vi "NewAutoWriteJSONFile.vi"(9 "Array":T2[](array[typedef]), 10 "Comment":string, 11 "Trajectory File Name":path) -> (0 "error out":errorcluster)   [LabVIEW 2023]
doc: "Create a CSV file from a Trajectory data structure. This can be used on a PC or the RoboRIO.\n\nParameters:\n - Trajectory - Data structure containing trajectory\n - TrajectoryConfig - Trajectory configuration\n - Trajectory File Name - File name to write to. Existing files are overwritten.\n - Comment - Comment string to include in file comments.\n - Waypoints - waypoints to include in file comments\n - TrajectoryIsRelative - Relative if TRUE otherwise absolute\n - TrajectoryIsCubic - Cubic if TRUE otherwise Quintic\n\nReturns:\n - Error out - returned error cluster\n\nReturns:\n - outTrajectory - Trajectory data structure\n - Error out - returned error cluster"
uses:
  NewAutoStepTypedef.ctl
  NewAutoStepTypeEnum.ctl
  <vilib>/Rock Robotics/WPI/ThirdParty/JAS_Junk/TrajLib/Trajectory_Library.lvlib
panel:
  out "AutoRoutine":T1
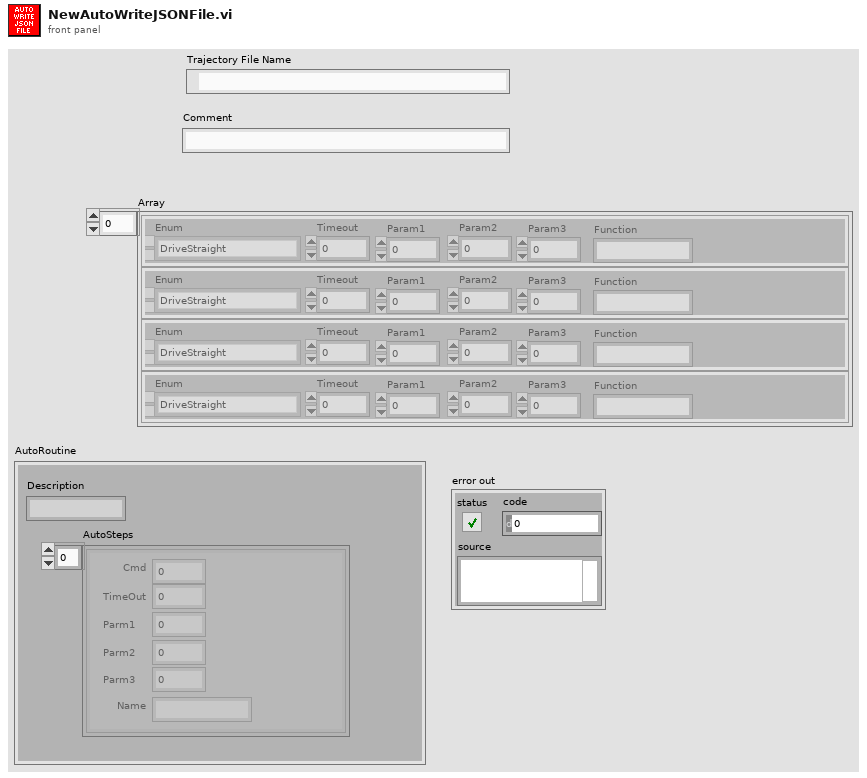
[diagram p1: front panel]
types:
  T1 = cluster{"Description":string, "AutoSteps":cluster{"Cmd":i32, "TimeOut":dbl, "Parm1":dbl, "Parm2":dbl, "Parm3":dbl, "Name":string}[]}
  T2 = typedef "NewAutoStepTypedef.ctl" = cluster{"Enum":T3, "Timeout":dbl, "Param1":dbl, "Param2":dbl, "Param3":dbl, "Function":string}
  T3 = typedef "NewAutoStepTypeEnum.ctl" = enum16{"DriveStraight", "DriveTurn", "FollowAbsoluteTrajectory", "FollowRelativeTrajectory", "AutoWait", "ElevToRest", "ElevToFloor", "ElevToSource", "ElevToL1", "ElevToL2", "ElevToL3", "ElevToL4", "ElevToAlgae1", "ElevToAlgae2", "ElevToBarge", "ElevCancel", "IntakeCoral", "IntakeAlgae", "IntakeDepositCoral", "IntakeDepositAlgae", "IntakeCancel", "ElevRestWait", "ElevFloorWait", "ElevSourceWait", "ElevL1Wait", "ElevL2Wait", "ElevAlgae1Wait", "ElevL3Wait", "ElevAlgae2Wait", "ElevL4Wait", "ElevBargeWait", "IntakeWait", "FollowAbsTrajWithTimedCmd", "FollowRelTrajWithTimedCmd"}
  T4 = cluster{"Cmd":i32, "TimeOut":dbl, "Parm1":dbl, "Parm2":dbl, "Parm3":dbl, "Name":string}
  T5 = enum16{"open", "replace", "create", "open or create", "replace or create", "replace or create with confirmation"}
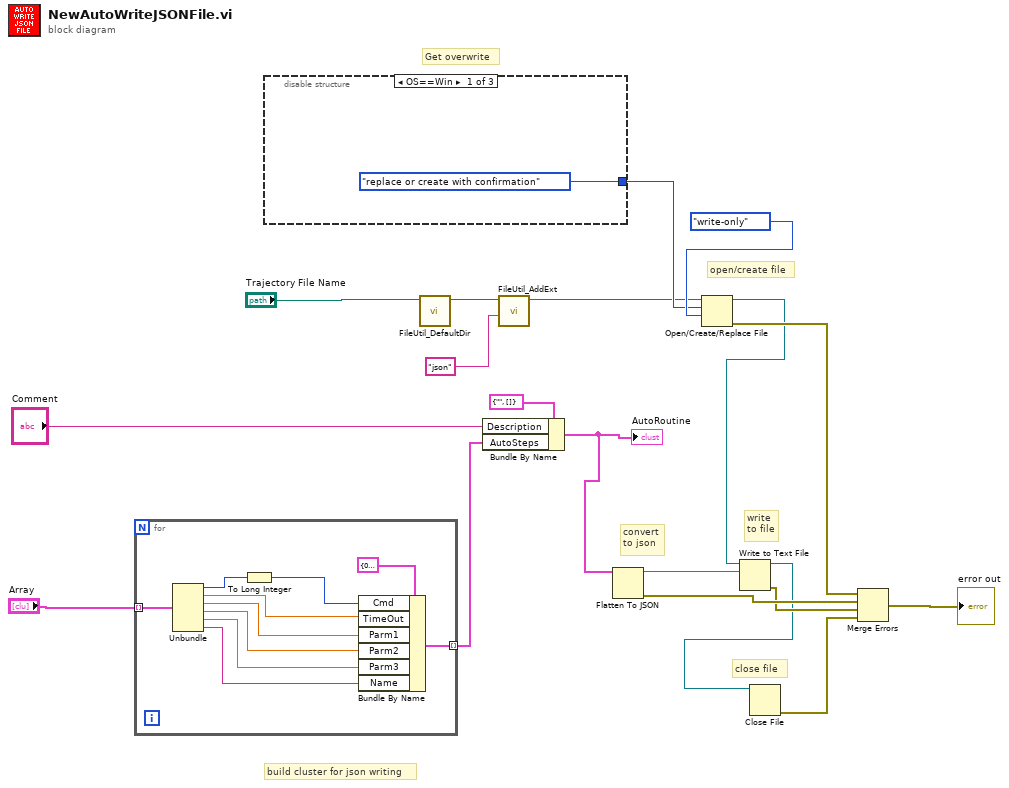
[diagram p0: block diagram]
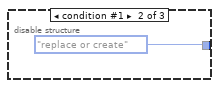
[diagram p2: hidden frame]
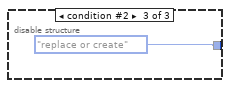
[diagram p3: hidden frame]
diagram:
  # "write\nto file"
  # "convert\nto json"
  # "build cluster for json writing"
  # "Get overwrite"
  # "open/create file"
  # "close file"
  n1 = for {
    tunnel: "Array" -> [w29] mode=indexing
    tunnel: [w20] -> w8 mode=indexing
    n2 = Unbundle(w29) -> ("Enum"=w28:T3, "Timeout"=w25:dbl, "Param1"=w24:dbl, "Param2"=w23:dbl, "Param3"=w22:dbl, "Function"=w21:string)
    n3 = To Long Integer(number=w28) -> (32bit integer=w26:i32)
    n4 = Bundle By Name(cluster=T4 {"Cmd"=0, "TimeOut"=0.0, "Parm1"=0.0, "Parm2"=0.0, "Parm3"=0.0, "Name"=""} ("AutoStep"), "Cmd"=w26, "TimeOut"=w25, "Parm1"=w24, "Parm2"=w23, "Parm3"=w22, "Name"=w21) -> (w20:T4)
  }
  n5 = disable-structure shown="OS==Win" {
    disable-tunnel: [T5."replace or create with confirmation" ("operation (0:open)") T5."replace or create" ("operation (0:open)") T5."replace or create" ("operation (0:open)")] -> w17
    frame condition #0 (active) {
    }
    frame condition #1 {
    }
    frame condition #2 {
    }
  }
  n6 = call <vilib>:"FileUtil_DefaultDir.vi"("Path in"="Trajectory File Name") -> ("Path Out"=w16:path)  [unwired: 10 in]
  n7 = Bundle By Name(cluster=T1 {"Description"="", "AutoSteps"=[]} ("AutoRoutine"), "Description"="Comment", "AutoSteps"=w8) -> (w7:T1)
  "AutoRoutine" <- w7
  n8 = call <vilib>:"FileUtil_AddExt.vi"("Extension"="json", "Path in"=w16) -> ("Path out"=w13:path)  [unwired: 9 in]
  n9 = Flatten To JSON(anything=w7) -> (JSON string=w6:string, 11:w5:errorcluster)  [unwired: 2 in]
  n10 = Open/Create/Replace File(file path (use dialog)=w13, operation (0:open)=w17, access (0:read/write)=enum16{"read/write", "read-only", "write-only"}."write-only") -> (refnum out=w9:refnum<file>, error out=w18:errorcluster)  [unwired: 3 in, 1 out]
  n11 = Write to Text File(file (use dialog)=w9, text=w6) -> (refnum out=w3:refnum<file>, error out=w4:errorcluster)  [unwired: 2 in, 1 out]
  n12 = Close File(refnum=w3) -> (error out=w2:errorcluster)  [unwired: 1 in, 1 out]
  n13 = Merge Errors(w18, w5, w4, w2) -> (→"error out":errorcluster)
